vi "test8-UserLog_Queue.vi"(8 "error in (no error)":errorcluster, 11 "TestCase in":refnum<class "testcase-CSMGlobalLog.lvclass">) -> (0 "error out":errorcluster, 3 "TestCase out":refnum<class "testcase-CSMGlobalLog.lvclass">)   [LabVIEW 2017, in "testcase-CSMGlobalLog.lvclass"]
uses:
  testcase-CSMGlobalLog.lvclass
  testcase-CSMGlobalLog.lvclass/testcase-CSMGlobalLog.ctl
  ed57623f-cc02-4141-adee-02d92d4e7552.vi
  src/user.lib/_NEVSTOP/Communicable State Machine(CSM)/_Support/GlobalEvent/GEvt-Generate with Rule Check.vi
  src/user.lib/_NEVSTOP/Communicable State Machine(CSM)/AdvanceAPI/CSM - Convert Error to Argument.vi
  src/user.lib/_NEVSTOP/Communicable State Machine(CSM)/_Support/GlobalEvent/Cache-GEvt Refs.vi
  src/user.lib/_NEVSTOP/Communicable State Machine(CSM)/AdvanceAPI/CSM - Make String Arguments Safe.vi
  src/user.lib/_NEVSTOP/Communicable State Machine(CSM)/_Support/ChangeFlag/FlagInstance-GEvt Refs.vi
  src/user.lib/_NEVSTOP/Communicable State Machine(CSM)/AdvanceAPI/CSM - Keywords.vi
  src/user.lib/_NEVSTOP/Communicable State Machine(CSM)/_Support/ChangeFlag/ChangeFlag-Read.vi
  src/user.lib/_NEVSTOP/Communicable State Machine(CSM)/_Support/ChangeFlag/ChangeFlagDB.vi
  src/user.lib/_NEVSTOP/Communicable State Machine(CSM)/_Support/GlobalEvent/FGV-GlobalEventRef(lvlibp).vi
  src/user.lib/_NEVSTOP/Communicable State Machine(CSM)/_Support/GlobalEvent/FGV-GlobalEventQueues(lvlibp).vi
  src/user.lib/_NEVSTOP/Communicable State Machine(CSM)/_Support/GlobalEvent/GEvt-Valid Subscribers.vi
  src/user.lib/_NEVSTOP/Communicable State Machine(CSM)/_Support/GlobalEvent/LogFilter/LogFilter - Check.vi
  src/user.lib/_NEVSTOP/Communicable State Machine(CSM)/_Support/GlobalEvent/LogFilter/LogFilter.lvclass
  <vilib>/addons/_JKI Toolkits/VI Tester/TestCase.llb/TestCase.lvclass
  src/user.lib/_NEVSTOP/Communicable State Machine(CSM)/Communicable State Machine.lvlib
  src/user.lib/_NEVSTOP/Communicable State Machine(CSM)/Utility/Periodic String Filter Setting.ctl
  C:/Program Files (x86)/National Instruments/LabVIEW 2017/vi.lib/addons/_JKI Toolkits/VI Tester/TestCase.llb/TestCase.lvclass
panel:
  out "String cache total":string
  out "LoopCount":i32
  out "String Cache Each Loop":string
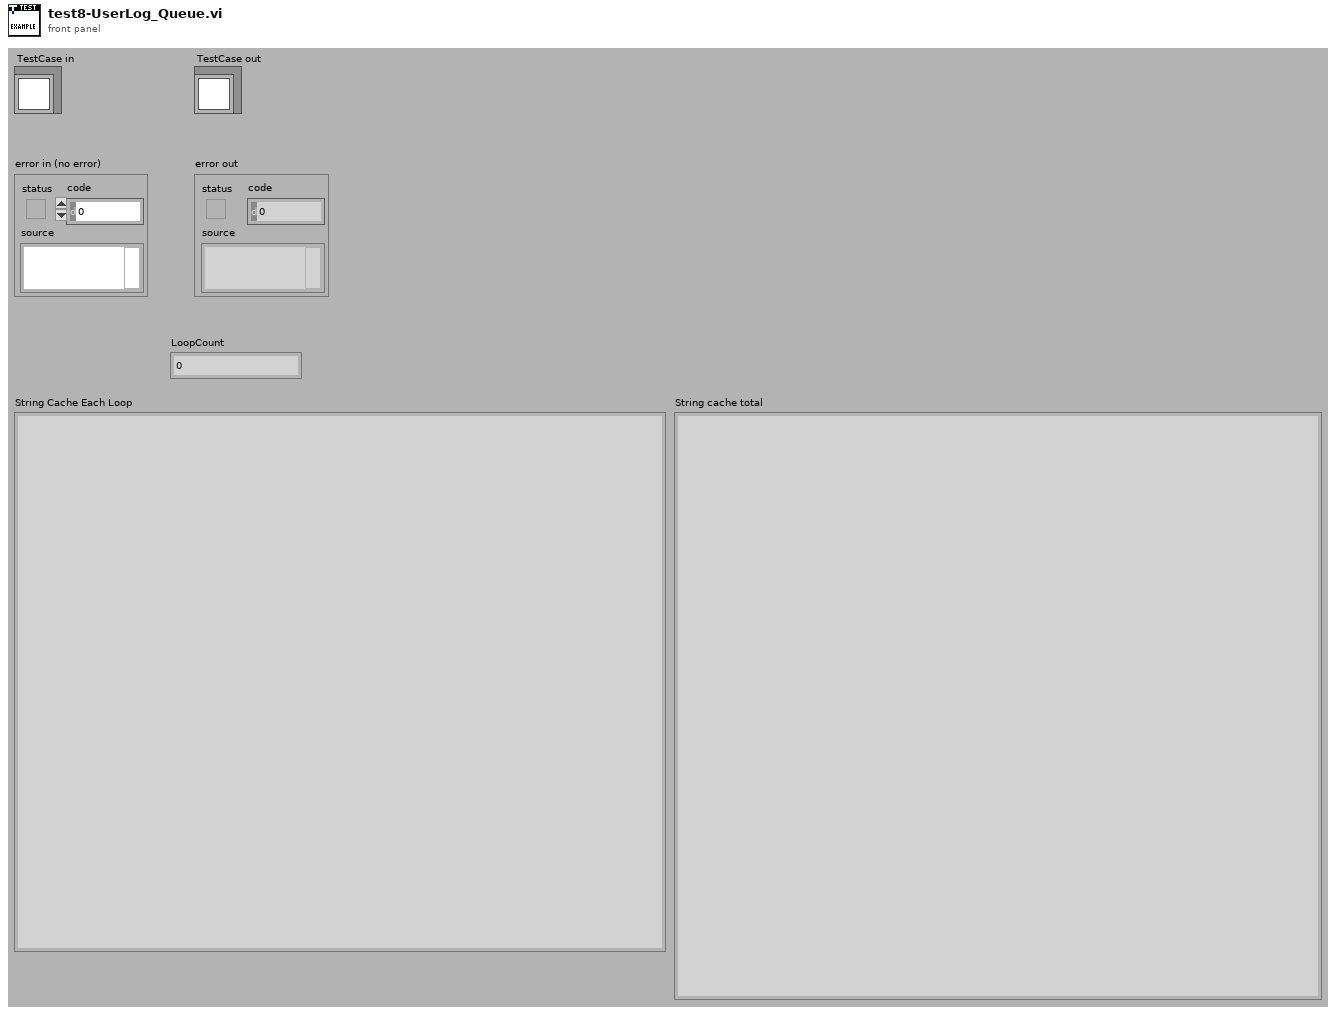
[diagram p1: front panel]
types:
  T1 = typedef "Communicable State Machine.lvlib/Periodic String Filter Setting.ctl" = cluster{"threashold(#/s)":dbl, "Check Peroid(s)":dbl}
  T2 = typedef "Communicable State Machine.lvlib/_CSM_GlobalLog_MSG.ctl" = cluster{"Name (\"\" to Use UUID)":string, "Current State":string, "Arguments":string, "Source Message":T3, "Source Module":string, "Complete(T)/Start(F)":bool, "LogType":T4, "Time Stamp":timestamp}
  T3 = typedef "Communicable State Machine.lvlib/_CSM_Response Source Message.ctl" = cluster{"‘State":string, "’Arguments":string, "’Error":errorcluster}
  T4 = typedef "Communicable State Machine.lvlib/_CSM_GlobalLog_MSG_TYPE.ctl" = enum16{"User Log", "State Change", "Status", "Interrupt", "Register", "Unregister", "Error Log", "Module Created", "Module Destroyed", "Async Message", "No-Rep Async Message", "Sync Message"}
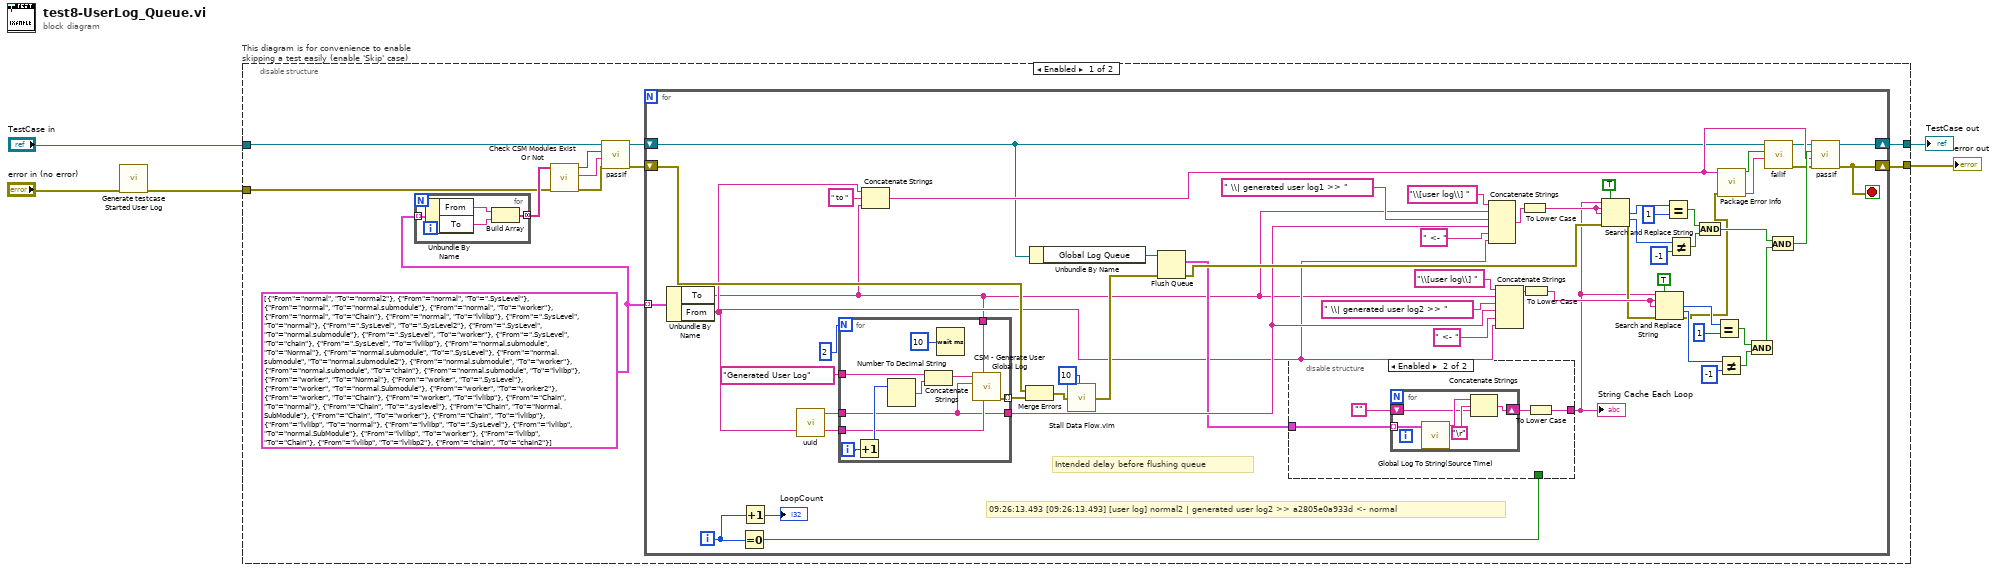
[diagram p0: block diagram]
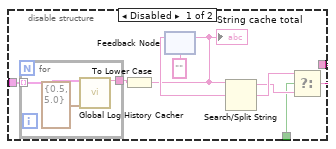
[diagram p2: hidden frame]
diagram:
  n1 = call "Generate testcase Started User Log.vi"("Error In"="error in (no error)") -> ("error out"=w1:errorcluster)  [unwired: 10 in]
  n2 = disable-structure "This diagram is for convenience to enable skipping a test easily (enable 'Skip' case)" shown="Enabled" {
    disable-tunnel: "TestCase in" -> [w9 w112]
    disable-tunnel: [w15 w110] -> w2
    disable-tunnel: [w16 w111] -> w4
    disable-tunnel: w1 -> [w7 w109]
    frame Enabled {
      w6 = cluster{"From":string, "To":string}[] [{"From"="normal", "To"="normal2"}, {"From"="normal", "To"=".SysLevel"}, {"From"="normal", "To"="normal.submodule"}, {"From"="normal", "To"="worker"}, {"From"="normal", "To"="Chain"}, {"From"="normal", "To"="lvlibp"}, {"From"=".SysLevel", "To"="normal"}, {"From"=".SysLevel", "To"=".SysLevel2"}, {"From"=".SysLevel", "To"="normal.submodule"}, {"From"=".SysLevel", "To"="worker"}, {"From"=".SysLevel", "To"="chain"}, {"From"=".SysLevel", "To"="lvlibp"}, {"From"="normal.submodule", "To"="Normal"}, {"From"="normal.submodule", "To"=".SysLevel"}, {"From"="normal.submodule", "To"="normal.submodule2"}, {"From"="normal.submodule", "To"="worker"}, {"From"="normal.submodule", "To"="chain"}, {"From"="normal.submodule", "To"="lvlibp"}, {"From"="worker", "To"="Normal"}, {"From"="worker", "To"=".SysLevel"}, {"From"="worker", "To"="normal.Submodule"}, {"From"="worker", "To"="worker2"}, {"From"="worker", "To"="Chain"}, {"From"="worker", "To"="lvlibp"}, {"From"="Chain", "To"="normal"}, {"From"="Chain", "To"=".syslevel"}, {"From"="Chain", "To"="Normal.SubModule"}, {"From"="Chain", "To"="worker"}, {"From"="Chain", "To"="lvlibp"}, {"From"="lvlibp", "To"="normal"}, {"From"="lvlibp", "To"=".SysLevel"}, {"From"="lvlibp", "To"="normal.SubModule"}, {"From"="lvlibp", "To"="worker"}, {"From"="lvlibp", "To"="Chain"}, {"From"="lvlibp", "To"="lvlibp2"}, {"From"="chain", "To"="chain2"}]
      n3 = for {
        tunnel: w6 -> [w20] mode=indexing
        tunnel: [w17] -> w13 mode=concatenating
        n4 = Unbundle By Name(w20) -> ("From"=w19:string, "To"=w18:string)
        n5 = Build Array(w19, w18) -> (w17:string[])
      }
      n6 = call "Check CSM Modules Exist Or Not.vi"("error in"=w7, "CSM names in"=w13) -> ("error out"=w11:errorcluster, "Debug string"=w12:string, "All Modules Exist?"=w14:bool)  [unwired: 7 in]
      n7 = call-dynamic "passIf.vi"("error in (no error)"=w11, "message (\"\")"=w12, "pass"=w14, "TestCase in"=w9) -> ("error out"=w8:errorcluster, "TestCase out"=w10:refnum<class "testcase-CSMGlobalLog.lvclass">)  [unwired: 6 in]
      n8 = for {
        shift-right: [w54] -> w16
        shift-left: w8 -> [w33]
        shift-right: [w77] -> w15
        shift-left: w10 -> [w23]
        tunnel: w6 -> [w43] mode=indexing
        i -> [w37]
        stop <- w54 stop-if-true
        # "Intended delay before flushing queue"
        # "09:26:13.493 [09:26:13.493] [user log] normal2 | generated user log2 >> a2805e0a933d <- normal"
        n9 = Unbundle By Name(w43) -> ("To"=w25:string, "From"=w26:string)
        n10 = Equal To 0?(x=w37) -> (x = 0?=w36:bool)
        n11 = Increment(x=w37) -> (x+1=→"LoopCount":i32)
        n12 = call "uuid.vi"() -> ("UUID"=w51:string)  [unwired: 11 in]
        n13 = for {
          N: 2 -> [_]
          tunnel: [w108] -> w34 mode=indexing
          tunnel: "Generated User Log" ("Log") -> [w107]
          tunnel: w51 -> [w100]
          tunnel: w25 -> [w102]
          tunnel: w26 -> [w101]
          tunnel: [w100] -> w42
          i -> [w104]
          n14 = Increment(x=w104) -> (x+1=w103:i32)
          n15 = Number To Decimal String(number=w103) -> (decimal integer string=w106:string)  [unwired: 1 in]
          n16 = Concatenate Strings(w107, w106) -> (w105:string)
          n17 = Wait (ms)(milliseconds to wait=u32 10) -> ()  [unwired: 1 out]
          n18 = call "CSM - Generate User Global Log.vi"("From Who"=w101, "Place (\"\" to Use VI's Name)"=w102, "Arguments"=w100, "Log"=w105) -> ("error out"=w108:errorcluster)  [unwired: 7 in]
        }
        n19 = Concatenate Strings(w26, " to " ("string"), w25) -> (w24:string)
        n20 = Merge Errors(w33, w34) -> (w32:errorcluster)
        n21 = Unbundle By Name(w23) -> ("Global Log Queue"=w76:refnum<queue>)
        n22 = call "Stall Data Flow.vim"("value in"=w32, "milliseconds to wait"=u32 10) -> ("value out"=w31:errorcluster)  [unwired: 1 out]
        n23 = Flush Queue(queue=w76, error in (no error)=w31) -> (remaining elements=w39:T2[], error out=w58:errorcluster)  [unwired: 1 out]
        n24 = disable-structure shown="Enabled" {
          disable-tunnel: [w80 w90] -> w38
          disable-tunnel: w36 -> [w79 _]
          disable-tunnel: w39 -> [w78 w92]
          frame Disabled {
            n25 = for {
              tunnel: w78 -> [w89] mode=indexing
              tunnel: [w88] -> w86
              n26 = call "Global Log History Cacher.vi"("Global Log Data"=w89, "Settings"=T1 {"threashold(#/s)"=0.5, "Check Peroid(s)"=5.0}) -> ("String Cache"=w88:string)  [unwired: 13 in]
            }
            n27 = To Lower Case(string=w86) -> (all lower case string=w81:string)
            "String cache total" <- w81
            n28 = feedback #1("") -> (w85:string)
            n29 = feedback-in #1(w81) -> ()
            n30 = Search/Split String(string=w81, search string/char (-)=w85) -> (substring before match=w82:string, match + rest of string=w83:string)  [unwired: 1 in, 1 out]
            n31 = Select(t=w83, s=w79, f=w82) -> (s? t:f=w80:string)
          }
          frame Enabled {
            n32 = for {
              tunnel: w92 -> [w98] mode=indexing
              shift-right: [w94] -> w91
              shift-left: "" -> [w95]
              n33 = call "Global Log To String(Source Time).vi"("Log"=w98) -> ("Log String"=w97:string)  [unwired: 9 in]
              n34 = Concatenate Strings(w97, "\r", w95) -> (w94:string)
            }
            n35 = To Lower Case(string=w91) -> (all lower case string=w90:string)
          }
        }
        "String Cache Each Loop" <- w38
        n36 = Concatenate Strings("\\[user log\\] " ("regular expression"), w25, " \\| generated user log1 >> " ("string"), w42, " <- " ("string"), w26) -> (w47:string)
        n37 = Concatenate Strings("\\[user log\\] " ("regular expression"), w25, " \\| generated user log2 >> " ("string"), w42, " <- " ("string"), w26) -> (w49:string)
        n38 = To Lower Case(string=w47) -> (all lower case string=w73:string)
        n39 = To Lower Case(string=w49) -> (all lower case string=w61:string)
        n40 = Search and Replace String(replace all?=TRUE ("replace all? (F)"), input string=w38, search string=w73, replace string=w73, error in=w58) -> (number of replacements=w72:i32, offset past replacement=w71:i32, error out=w60:errorcluster)  [unwired: 3 in, 1 out]
        n41 = Search and Replace String(replace all?=TRUE ("replace all? (F)"), input string=w38, search string=w61, replace string=w61, error in=w60) -> (number of replacements=w63:i32, offset past replacement=w64:i32, error out=w28:errorcluster)  [unwired: 3 in, 1 out]
        n42 = Equal?(x=w72, y=1) -> (x = y?=w69:bool)
        n43 = Not Equal?(x=w71, y=-1) -> (x != y?=w68:bool)
        n44 = And(x=w69, y=w68) -> (x .and. y?=w55:bool)
        n45 = Equal?(x=w63, y=1) -> (x = y?=w66:bool)
        n46 = call "Package Error Info.vi"("error in"=w28, "String in"=w24) -> ("packed error info out"=w29:string, "error status"=w30:bool)  [unwired: 8 in]
        n47 = Not Equal?(x=w64, y=-1) -> (x != y?=w67:bool)
        n48 = And(x=w66, y=w67) -> (x .and. y?=w59:bool)
        n49 = call-dynamic "failIf.vi"("message (\"\")"=w29, "fail"=w30, "TestCase in"=w23) -> ("error out"=w21:errorcluster, "TestCase out"=w22:refnum<class "testcase-CSMGlobalLog.lvclass">)  [unwired: 7 in]
        n50 = And(x=w55, y=w59) -> (x .and. y?=w35:bool)
        n51 = call-dynamic "passIf.vi"("error in (no error)"=w21, "message (\"\")"=w24, "pass"=w35, "TestCase in"=w22) -> ("error out"=w54:errorcluster, "TestCase out"=w77:refnum<class "testcase-CSMGlobalLog.lvclass">)  [unwired: 6 in]
      }
    }
    frame Disabled {
      # "skip test result while test is under development"
      n52 = call <vilib>:"skip.vi"("error in (no error)"=w109, "TestCase in"=w112) -> ("error out"=w111:errorcluster, "TestCase out"=w110:refnum<class "testcase-CSMGlobalLog.lvclass">)  [unwired: 8 in]
    }
  }
  "error out" <- w4
  "TestCase out" <- w2
